vi "ExeCmd_sync.vi"(4 "HighPrio":bool, 6 "CmdVIRef":refnum<vi>, 8 "ErrorIn":errorcluster, 9 "NameOfVi2Call(optional)":string, 10 "CmdData":variant, 11 "YActorIn":refnum<class "YActor.lvclass">) -> (0 "ErrorOut":errorcluster, 2 "ReplyData":variant, 3 "YActorOut":refnum<class "YActor.lvclass">)   [LabVIEW 2021, in "YActor.lvclass"]
uses:
  YActor.lvclass
  YActor.lvclass/YActor.ctl
  private/CallMode.ctl
  private/CmdCtrl.ctl
  AsyncErrorHandling.ctl
  private/VINameProperty.vi
  InlineReferencePool.vi
panel:
  # "Do not use this VI in a loop where different Cmd VI references are routed.\nThis will cause the execution of the first called command VI only"
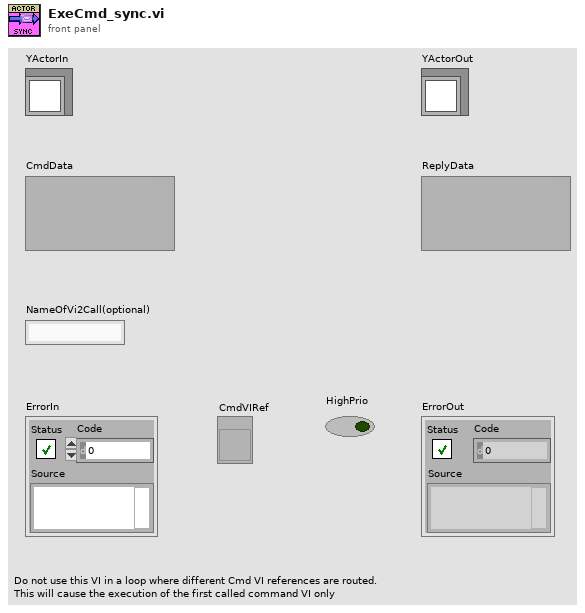
[diagram p1: front panel]
types:
  T1 = typedef "YActor.lvclass/CallMode.ctl" = enum16{"Standard", "Call&Collect"}
  T2 = typedef "YActor.lvclass/CmdCtrl.ctl" = cluster{"CmdData":variant, "CommandVI":string, "ReplyQ":i64, "Error":errorcluster, "Msg#":u32, "AsyncErrorHandling":T3, "CallMode":T1, "Source":string}
  T3 = typedef "YActor.lvclass/AsyncErrorHandling.ctl" = enum16{"Return after executing sync command", "Return before executing sync command", "Don't return error"}
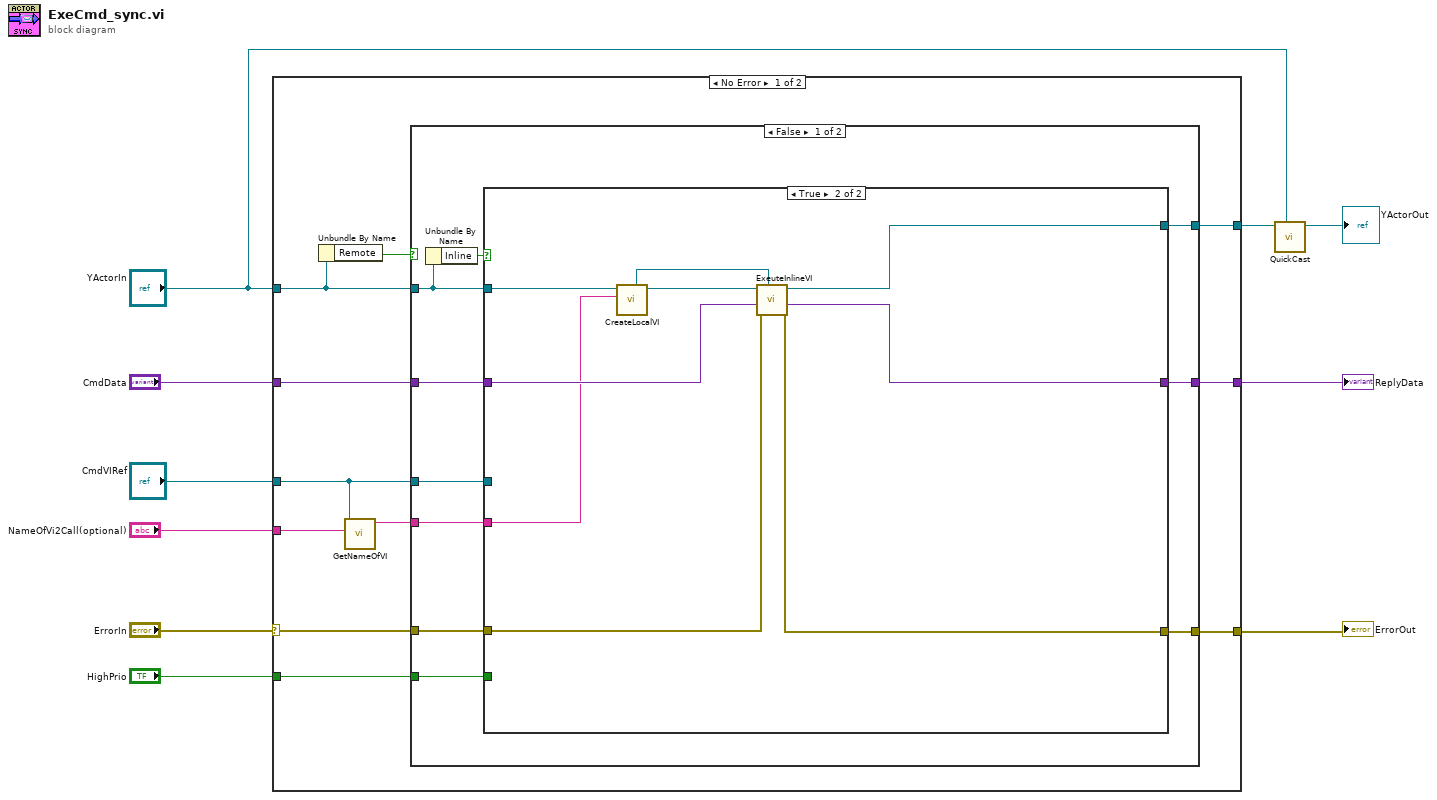
[diagram p0: block diagram]
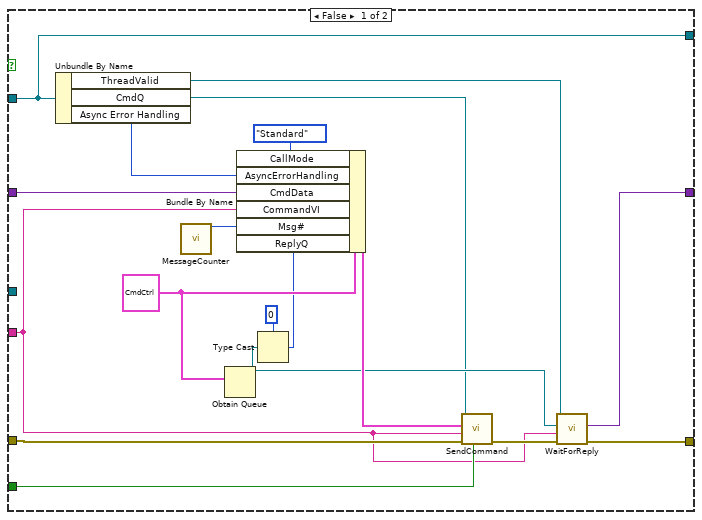
[diagram p2: hidden frame]
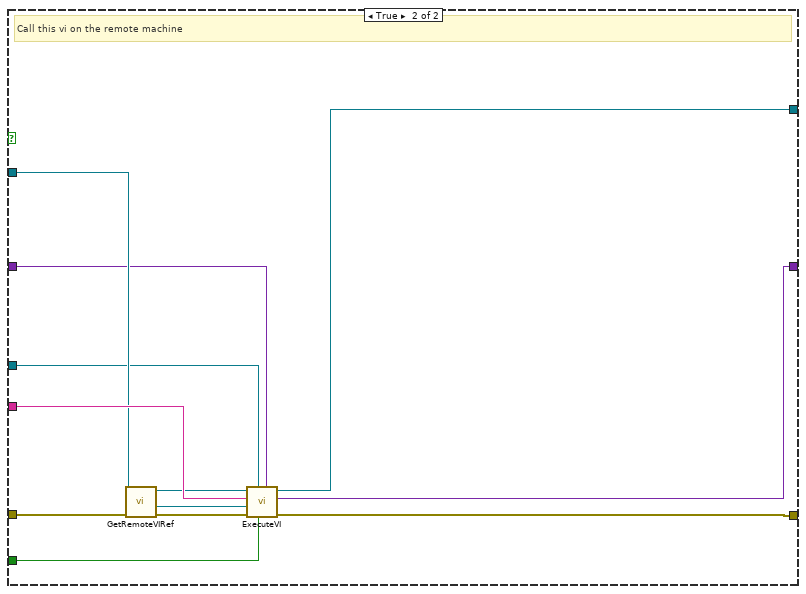
[diagram p3: hidden frame]
diagram:
  n1 = case shown="No Error" "ErrorIn" {
    selector: "ErrorIn" -> [w20 w73]
    tunnel: [w21 w73] -> w9
    tunnel: "YActorIn" -> [w11 w71]
    tunnel: "CmdData" -> [w17 w72]
    tunnel: "CmdVIRef" -> [w14 _]
    tunnel: [w19 w72] -> w1
    tunnel: "HighPrio" -> [w18 _]
    tunnel: [w16 w71] -> w4
    tunnel: "NameOfVi2Call(optional)" -> [w12 _]
    frame No Error {
      n2 = Unbundle By Name(w11) -> ("Remote"=w15:bool)
      n3 = call "GetNameOfVI.vi"("NameOfVi2Call(optional)"=w12, "VIIn"=w14) -> ("Name"=w13:string)  [unwired: 9 in]
      n4 = case shown="False" w15 {
        tunnel: [w29 w66] -> w19
        tunnel: [w31 w68] -> w21
        tunnel: w20 -> [w30 w70]
        tunnel: w18 -> [w28 w67]
        tunnel: w17 -> [w27 w61]
        tunnel: w14 -> [w26 w62]
        tunnel: w11 -> [w25 w63]
        tunnel: [w23 w60] -> w16
        tunnel: w13 -> [w22 w64]
        frame False {
          n5 = Unbundle By Name(w25) -> ("Inline"=w24:bool)
          n6 = case shown="True" w24 {
            tunnel: [w35 w51] -> w29
            tunnel: [w47 w57] -> w31
            tunnel: w30 -> [w49 w58]
            tunnel: w28 -> [w37 _]
            tunnel: w27 -> [w41 w56]
            tunnel: w26 -> [_ _]
            tunnel: w25 -> [w38 w52]
            tunnel: [w38 w55] -> w23
            tunnel: w22 -> [w36 w54]
            frame False {
              w46 = T2 {"CmdData"=variant(refnum<class> refnum), "CommandVI"="", "ReplyQ"=0, "Error"={"Status"=FALSE, "Code"=0, "Source"=""}, "Msg#"=0, "AsyncErrorHandling"=enum."Return after executing sync command", "CallMode"=enum."Standard", "Source"=""} ("CmdCtrl")
              n7 = Unbundle By Name(w38) -> ("ThreadValid"=w42:refnum<queue>, "CmdQ"=w43:refnum<queue>, "Async Error Handling"=w39:T3)
              n8 = call "MessageCounter.vi"() -> ("Msg#"=w34:u32)  [unwired: 11 in]
              n9 = Obtain Queue(element data type=w46) -> (queue out=w44:refnum<queue>)  [unwired: 4 in, 2 out]
              n10 = Type Cast(type=i64 0, x=w44) -> (*(type *) &x=w33:i64)
              n11 = Bundle By Name(cluster=w46, "CallMode"=CallMode."Standard", "AsyncErrorHandling"=w39, "CmdData"=w41, "CommandVI"=w36, "Msg#"=w34, "ReplyQ"=w33) -> (w45:T2)
              n12 = call "SendCommand.vi"("HighPrio"=w37, "ErrorIn"=w49, "Name"=w36, "CmdCtrl"=w45, "QueueIn"=w43) -> ("ErrorOut"=w48:errorcluster)  [unwired: 6 in]
              n13 = call "WaitForReply.vi"("ErrorIn"=w48, "Name"=w36, "ReplyQueue"=w44, "Alive"=w42) -> ("ErrorOut"=w47:errorcluster, "Reply"=w35:variant)  [unwired: 6 in]
            }
            frame True {
              n14 = call "CreateLocalVI.vi"("Name"=w54, "YActorIn"=w52) -> ("YActorOut"=w53:refnum<class "YActor.lvclass">, "CreatedVI"=w50:refnum<vi>)  [unwired: 8 in]
              n15 = call "ExeuteInlineVI.vi"("CreatedVI"=w50, "ErrorIn"=w58, "CmdData"=w56, "YActorIn"=w53) -> ("ErrorOut"=w57:errorcluster, "ReplyData"=w51:variant, "YActorOut"=w55:refnum<class>)  [unwired: 5 in]
            }
          }
        }
        frame True {
          # "Call this vi on the remote machine"
          n16 = call "GetRemoteVIRef.vi"("ErrorIn"=w70, "YActorIn"=w63) -> ("ErrorOut"=w69:errorcluster, "CreatedVI"=w65:refnum<vi>, "YActorOut"=w59:refnum<class "YActor.lvclass">)  [unwired: 7 in]
          n17 = call "ExecuteVI.vi"("CmdData"=w61, "HighPrio"=w67, "CmdVIRef"=w62, "ErrorIn"=w69, "VIToExecute"=w65, "Name"=w64, "YActorIn"=w59) -> ("ErrorOut"=w68:errorcluster, "ReplyData"=w66:variant, "YActorOut"=w60:refnum<class "YActor.lvclass">)  [unwired: 2 in]
        }
      }
    }
    frame Error {
    }
  }
  "ErrorOut" <- w9
  "ReplyData" <- w1
  n18 = call "QuickCast.vi"("YActor in"=w4, "object target type"="YActorIn") -> ("object out"=→"YActorOut":refnum<class "YActor.lvclass">)  [unwired: 9 in]
